vi "THz_TimeDelay.vi"(8 "error in (no error)":errorcluster, 11 "Transport":refnum<class "SMO.Transport.lvclass">) -> (0 "error out":errorcluster, 3 "Transport out":refnum<class "SMO.Transport.lvclass">)   [LabVIEW 2019, in "SMO.Transport.lvclass"]
uses:
  SMO.Transport.lvclass
  <userlib>/LevyLab/Instrument Framework/Instrument Types/Cryostat/Instrument.Cryostat.lvclass
  Control Experiment/Control Experiment.lvclass
  <userlib>/LevyLab/Krohn Hite 7008/Instrument.KH7008.lvclass
  <userlib>/LevyLab/Lockin-Multichannel/Instrument.Lockin/Instrument.Lockin.lvclass
  Control Experiment/Typedefs/Instruments--cluster.ctl
  <userlib>/LevyLab/Instrument Framework/Instrument Types/VSource/Instrument.VSource.lvclass
  <userlib>/LevyLab/Instrument Framework/Instrument Types/VNA/Instrument.VNA.lvclass
  <userlib>/LevyLab/Instrument Framework/Instrument Types/Strain/Instrument.Strain.lvclass
  <userlib>/LevyLab/Instrument Framework/Instrument Types/CBridge/Instrument.CBridge.lvclass
  <vilib>/measure/NI_MAPro.lvlib
  <userlib>/LevyLab/XY Utilities/xy_utilities.lvlib
  <userlib>/LevyLab/XY Utilities/subVIs/Waveform to XY (single).vi
  <userlib>/LevyLab/XY Utilities/subVIs/Get X and Y (single).vi
  <vilib>/measure/maspectr.llb/FFT Power Spectrum and PSD for 1 Chan.vi
  <vilib>/Waveform/WDTOps.llb/WDT Append Waveforms DBL.vi
  <userlib>/_MGI/Timing/MGI Wait/MGI Wait (U32).vi
  <userlib>/LevyLab/Lockin-Multichannel/Instrument.DAQ/Typedefs/Set State-enum.ctl
  <userlib>/LevyLab/Lockin-Multichannel/Instrument.DAQ/Instrument.DAQ.lvclass
  <userlib>/LevyLab/Instrument Framework/Instrument Types/Delay Line/Instrument.DelayLine.lvclass
  SMO.Control Experiment/SMO.Control Experiment.lvclass
  C:/Program Files (x86)/National Instruments/LabVIEW 2019/user.lib/LevyLab/Instrument Framework/SMOs/Instrument/Instrument.lvclass
  C:/Program Files (x86)/National Instruments/LabVIEW 2019/vi.lib/JKI/JKI SMO/SMO/SMO.lvclass
  <vilib>/measure/maresamp.llb/Resample Pair of Arrays (single shot).vi
panel:
  out "Horizontal Progress Bar":dbl(slide)=0.5013000000000001 scale=-0.5..0.5
  out "Signal vs Time":T1(graph)
  out "Delay vs Time":cluster{"Time":dbl[], "Delay":dbl[]}(graph)
  out "Power Spectrum":cluster{"f0":dbl, "df":dbl, "magnitude":dbl[]}[](graph) caption="Power spectrum of time domain signal"
  in  "stop":bool
  in  "Experiment Comments":string="describe only the experiment you're doing right now"
  in  "Experiment Folder":string="05 - folder name"
  out "Delay (ps)":dbl
  out "Elapsed Time (s)":u32
  out "T (mK)":dbl
  out "Refresh Time (ms)":u32
  in  "Sweep Time (s)":dbl=10.0 format="%#_3p"
  in  "Initial Wait (s)":u32=1
  in  "Delay End (ps)":dbl=0.5
  in  "Delay Start (ps)":dbl=-0.5
  in  "Fs (S/s)":dbl=1000.0 min=1000.0 max=204800.0 format="%#_13g"
  in  "Lockin Refresh (s)":dbl=2.0
  in  "Timeout (ms)":i32=1000
  out "Current State":string="Exit"
  # "Start"
  # "End"
  # "*** Folder and comments are only read if this VI is top level. If is is called from Sweep Control then the folder and comments come from Sweep Control.vi ***"
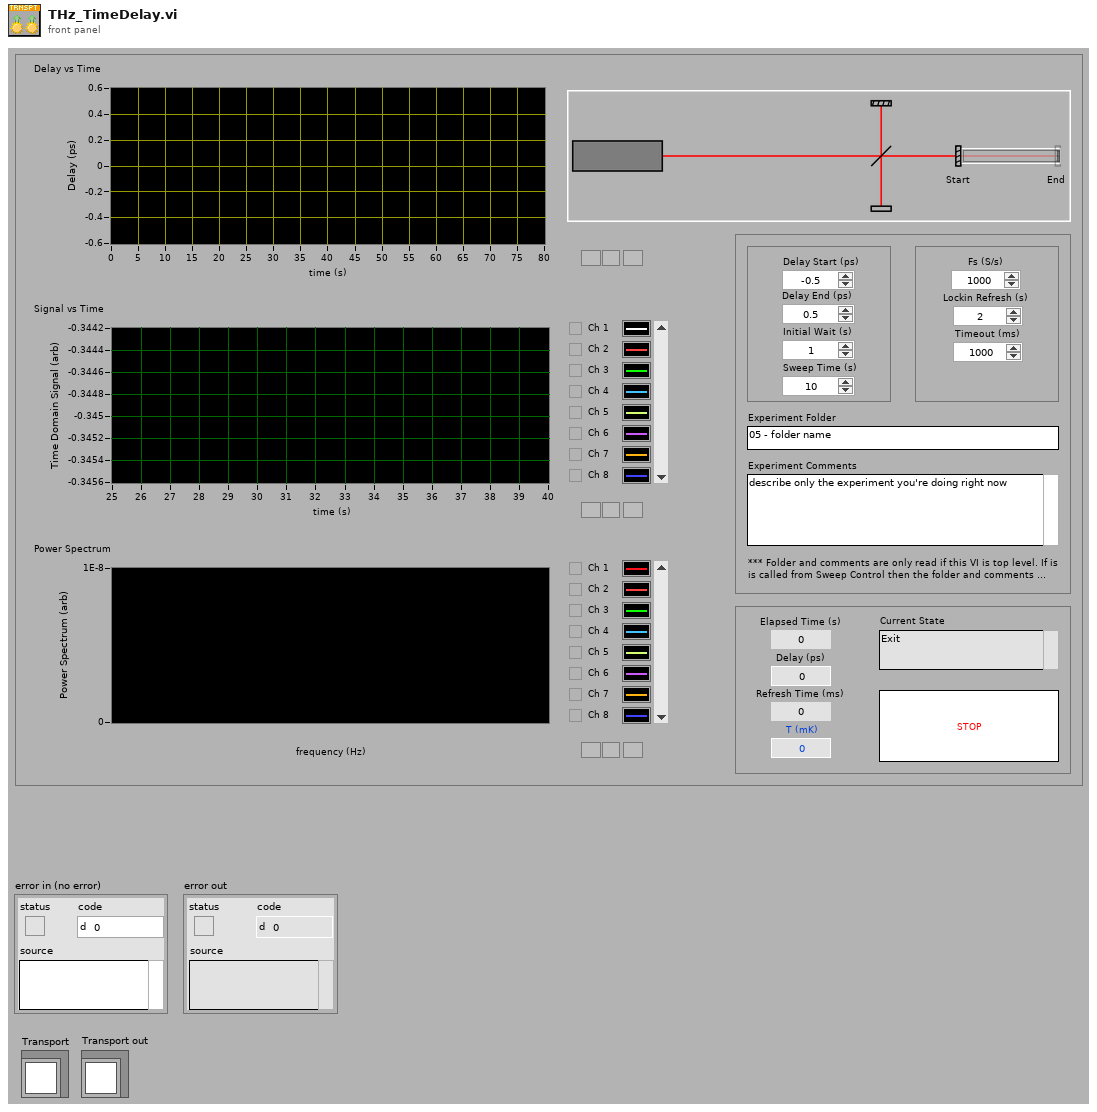
[diagram p1: front panel]
types:
  T1 = cluster{"Delay Start (ps)":dbl, dbl, "Y":dbl[]}[]
  T2 = enum32{"Invalid", "Standard", "Closed", "Hidden", "Minimized", "Maximized"}
  T3 = enum32{"invalid app kind", "Development System", "Run Time System", "Student Edition", "Embedded LabVIEW", "Evaluation", "Custom"}
  T4 = typedef "Lockin.DAQ.lvclass/State-enum.ctl" = enum16{"idle", "created", "started", "stopped", "sweeping"}
  T5 = typedef "Control Experiment.lvclass/Instruments--cluster.ctl" = cluster{"KH7008":refnum<class "Instrument.KH7008.lvclass">[], "Lockin":refnum<class "Instrument.Lockin.lvclass">, "Temperature":refnum<class "Instrument.Cryostat.lvclass">, "Magnet":refnum<class "Instrument.Cryostat.lvclass">, "Rotator":refnum<class "Instrument.Cryostat.lvclass">, "Level":refnum<class "Instrument.Cryostat.lvclass">, "Capacitance Bridge":refnum<class "Instrument.CBridge.lvclass">, "Delay Line":refnum<class "Instrument.DelayLine.lvclass">, "Strain Cell":refnum<class "Instrument.Strain.lvclass">, "VNA":refnum<class "Instrument.VNA.lvclass">, "Voltage Source":refnum<class "Instrument.VSource.lvclass">}
  T6 = cluster{"Core":cluster{"Current VI Reference":refnum<vi>, "Close Panel on Exit?":bool}, "Transport":refnum<class "SMO.Transport.lvclass">, "Control Experiment":refnum<class "SMO.Control Experiment.lvclass">, "Instruments":T5, "Elapsed Time":dbl[], "Absolute Time":dbl[], "Temperature":dbl, "Magnet":dbl, "Delay":dbl[], "AI Waveform (s)":waveform(dbl)[], "AI Waveform (ps)":waveform(dbl)[], "t0":timestamp, "Sweep Value":dbl[], "ms [0]":u32, "ms [i]":u32, "Delay Range (ps)":dbl, "Delay Speed (ps/s)":dbl, "reset":bool, "delay line finish?":bool, "Execution:State":enum32{"Bad", "Idle", "Run top level", "Running"}}
  T7 = enum32{"Bad", "Idle", "Run top level", "Running"}
  T8 = cluster{"Current VI Reference":refnum<vi>, "Close Panel on Exit?":bool}
  T9 = typedef "Instrument.DAQ.lvclass/Get State-enum.ctl" = enum16{"idle", "created", "started", "stopped", "sweeping"}
  T10 = typedef "Instrument.DAQ.lvclass/DAQ.Sampling.Sampling--Cluster.ctl" = cluster{"Fs":dbl, "#s":i32}
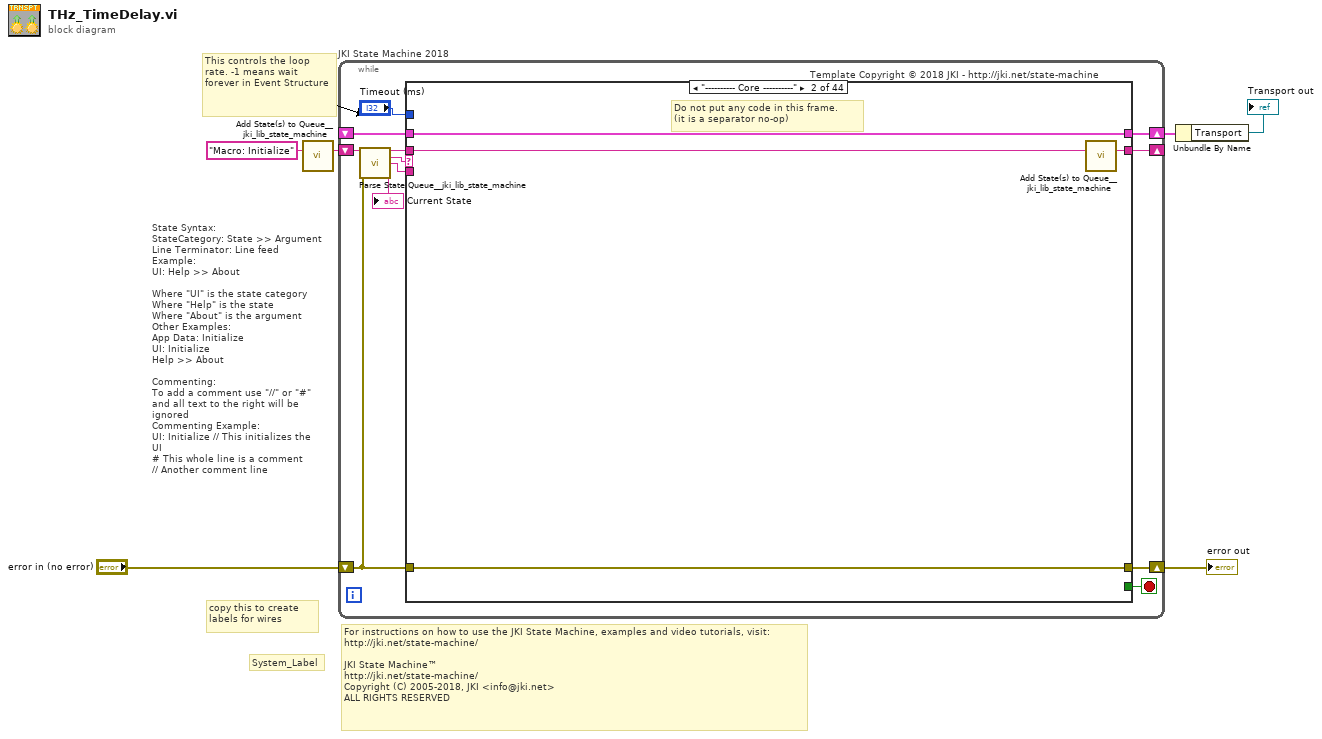
[diagram p0: block diagram]
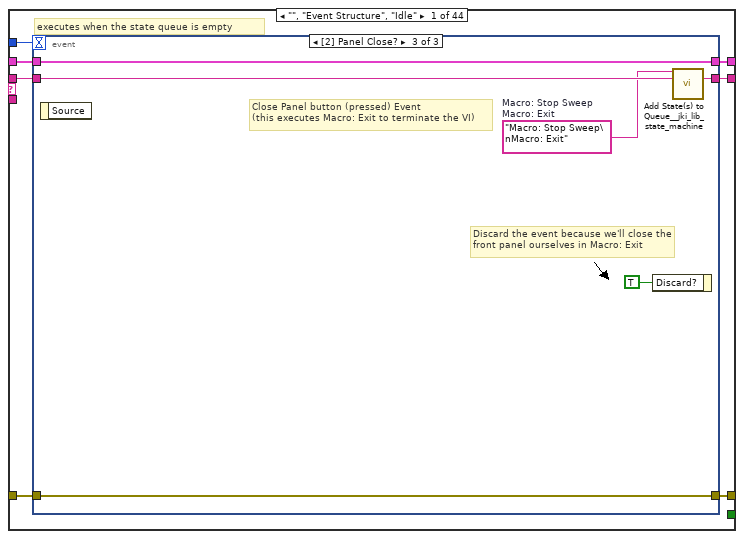
[diagram p2: hidden frame]
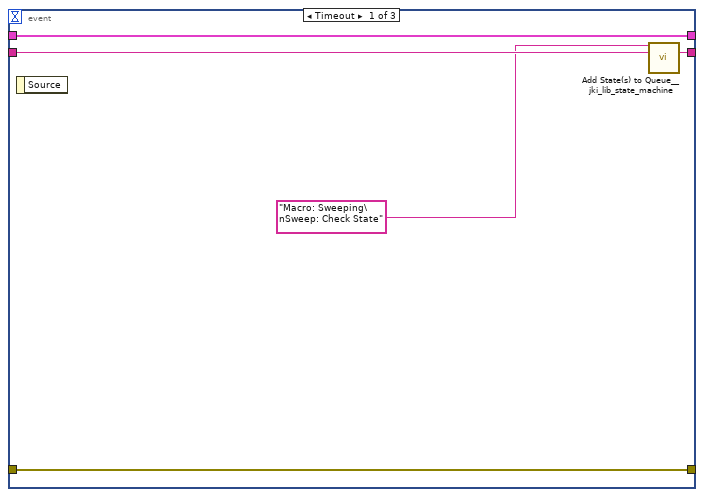
[diagram p3: hidden frame]
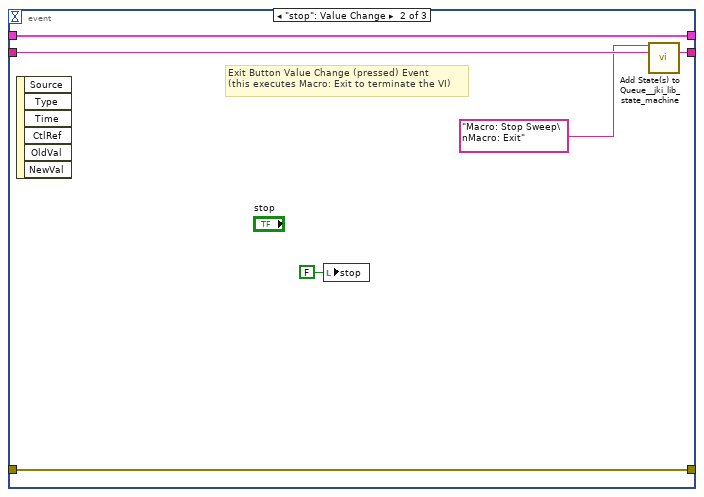
[diagram p4: hidden frame]
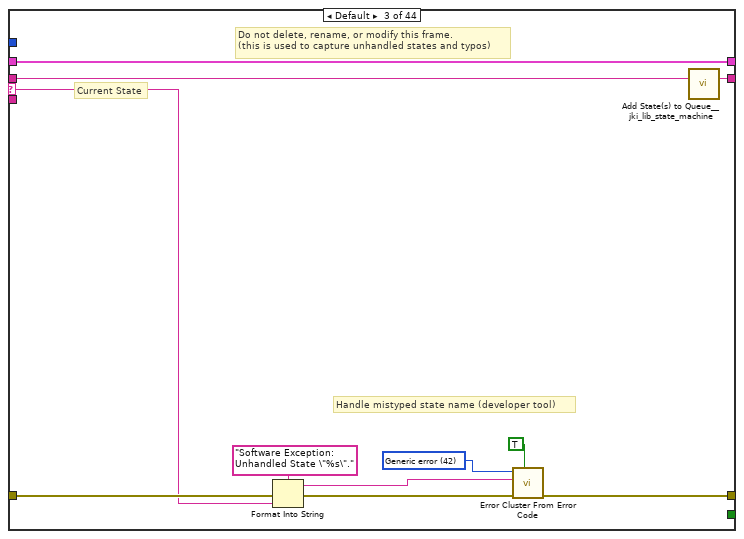
[diagram p5: hidden frame]
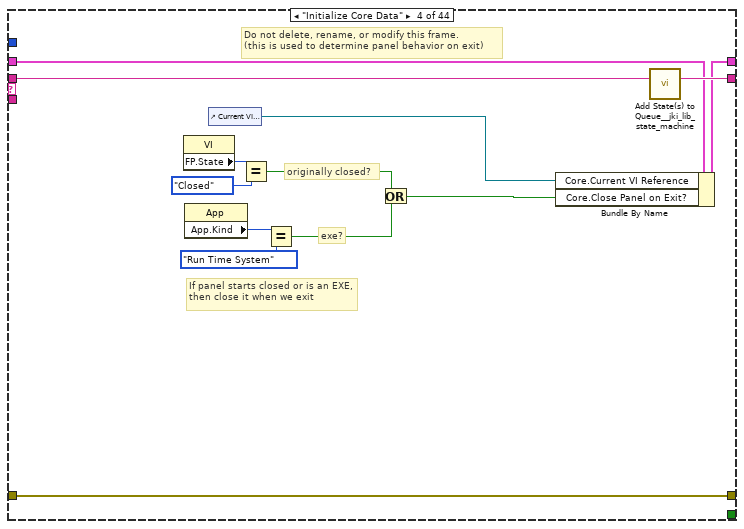
[diagram p6: hidden frame]
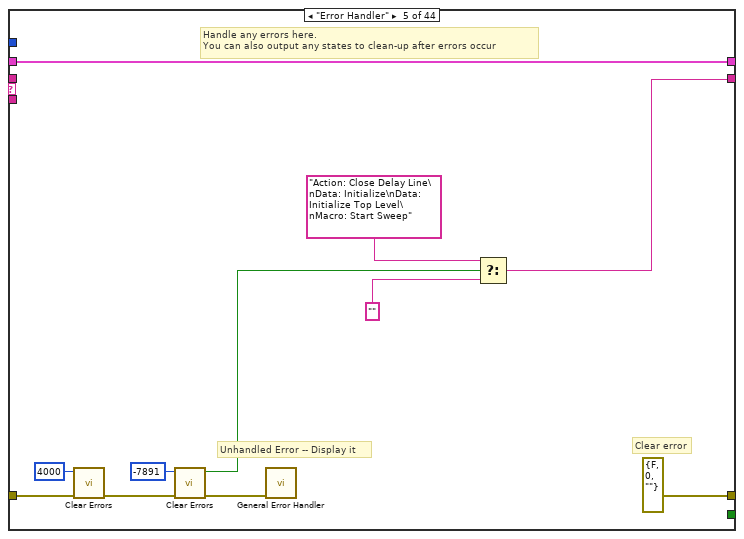
[diagram p7: hidden frame]
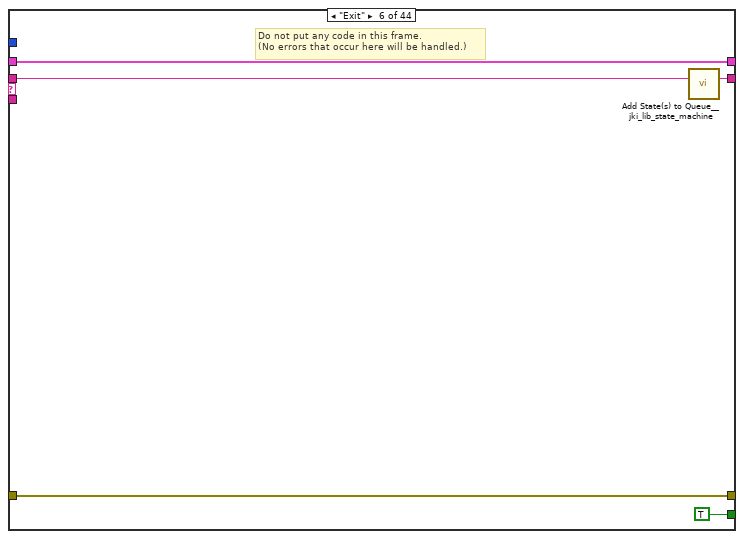
[diagram p8: hidden frame]
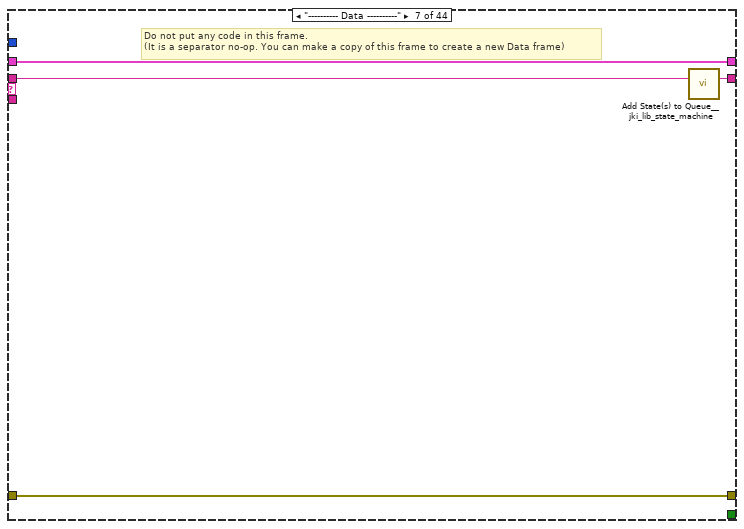
[diagram p9: hidden frame]
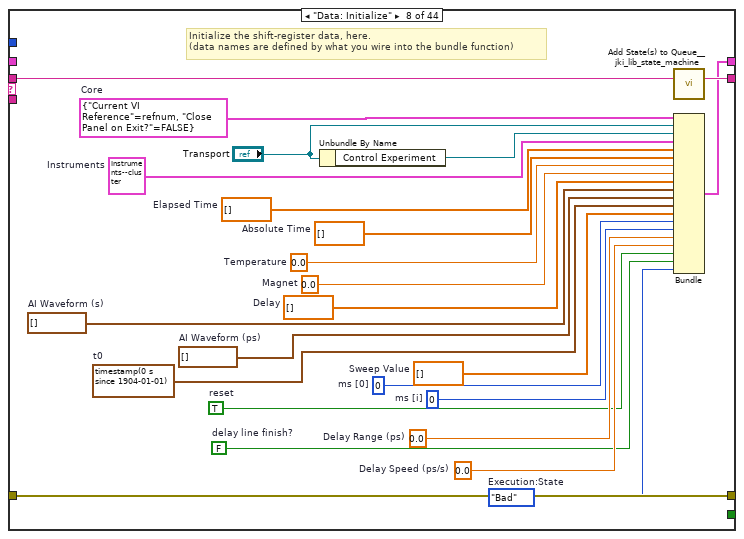
[diagram p10: hidden frame]
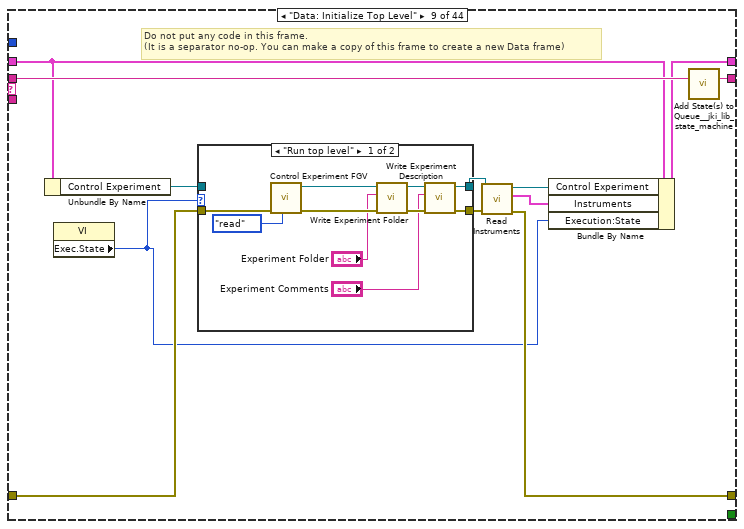
[diagram p11: hidden frame]
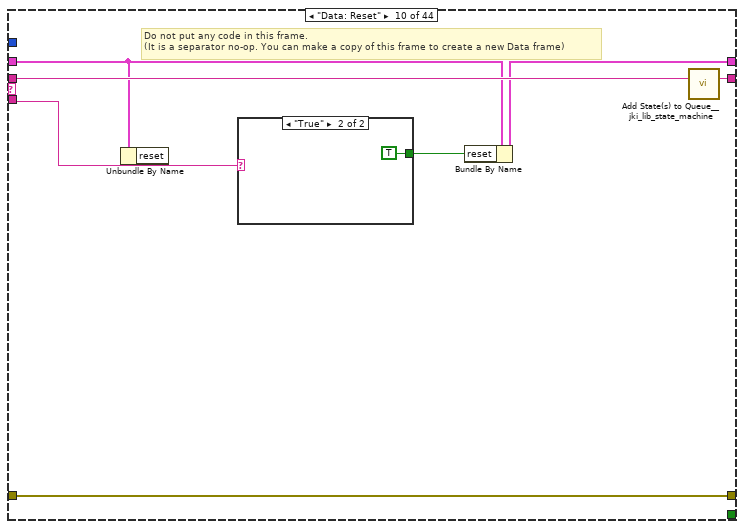
[diagram p13: hidden frame]
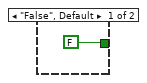
[diagram p14: hidden frame]
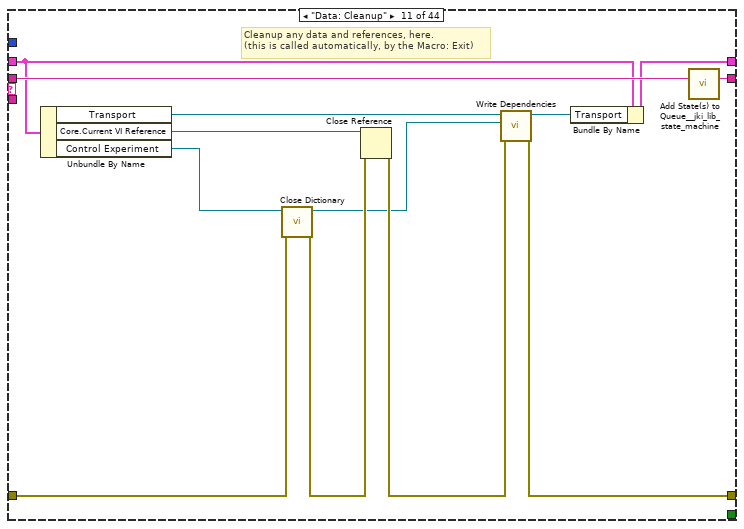
[diagram p15: hidden frame]
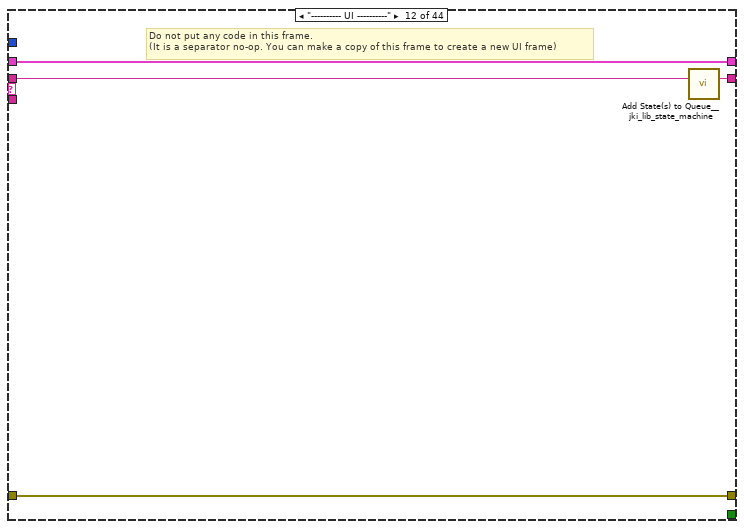
[diagram p16: hidden frame]
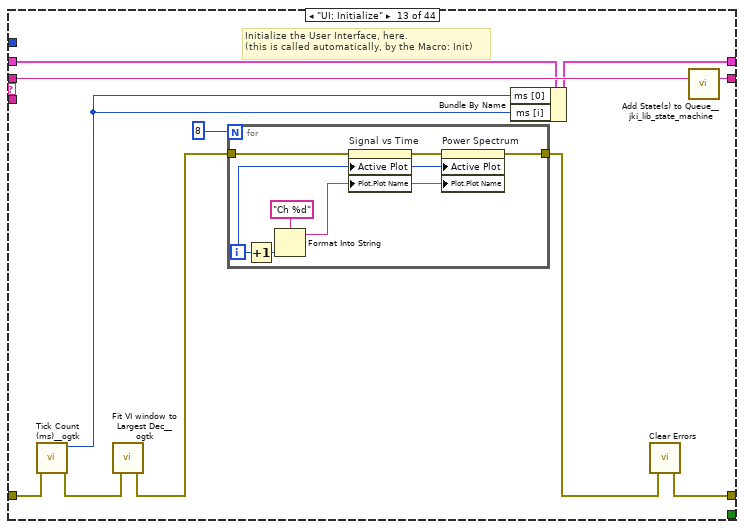
[diagram p17: hidden frame]
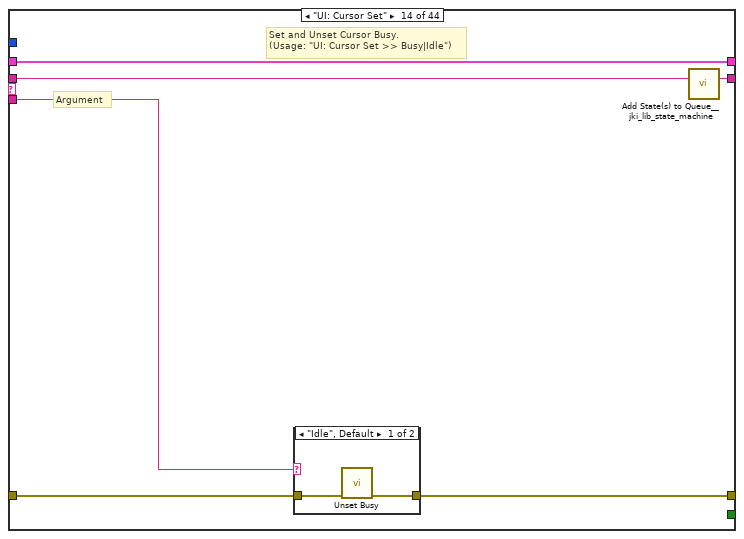
[diagram p18: hidden frame]
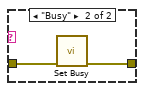
[diagram p19: hidden frame]
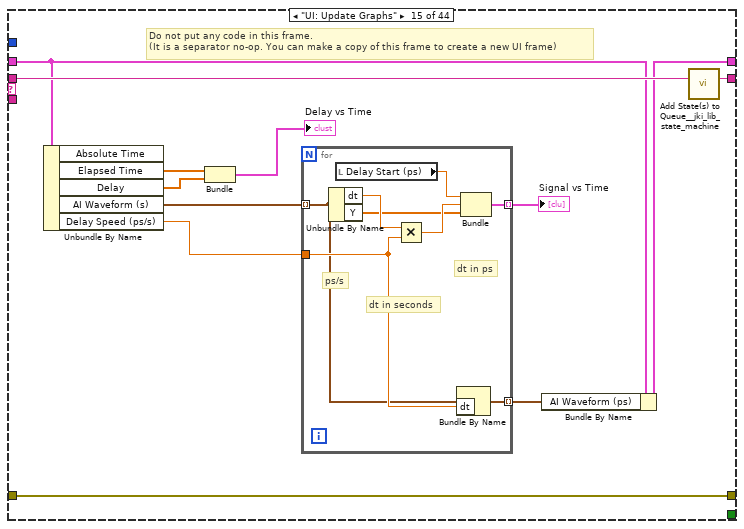
[diagram p20: hidden frame]
diagram:
  # "For instructions on how to use the JKI State Machine, examples and video tutorials, visit:\nhttp://jki.net/state-machine/\n\nJKI State Machine™\nhttp://jki.net/state-machine/\nCopyright (C) 2005-2018, JKI <info@jki.net>\nALL RIGHTS RESERVED"
  # "State Syntax:\nStateCategory: State >> Argument\nLine Terminator: Line feed\nExample:\nUI: Help >> About\n\nWhere \"UI\" is the state category\nWhere \"Help\" is the state\nWhere \"About\" is the argument\nOther Examples:\nApp Data: Initialize\nUI: Initialize\nHelp >> About\n\nCommenting:\nTo add a comment use \"//\" or \"#\" and all text to the right will be ignored\nCommenting Example:\nUI: Initialize // This initializes the UI\n# This whole line is a comment\n// Another comment line"
  # "copy this to create labels for wires"
  # "This controls the loop rate. -1 means wait forever in Event Structure"
  # "System_Label"
  n1 = call <vilib>:"Add State(s) to Queue__jki_lib_state_machine.vi"("State(s) in (\"\")"="Macro: Initialize") -> ("States Out"=w6:string)  [unwired: 14 in]
  n2 = while "JKI State Machine 2018" {
    shift-right: [w11] -> w4
    shift-left: _ -> [w10]
    shift-right: [w14] -> w3
    shift-left: "error in (no error)" -> [w8]
    shift-right: [w13] -> _
    shift-left: w6 -> [w15]
    stop <- w12 stop-if-true
    # "Template Copyright © 2018 JKI - http://jki.net/state-machine"
    n3 = call <vilib>:"Parse State Queue__jki_lib_state_machine.vi"("State Queue"=w15, "Error In (no error)"=w8) -> ("Remaining States"=w17:string, "Current State"=w7:string, "Arguments"=w16:string)  [unwired: 11 in]
    "Current State" <- w7
    n4 = case shown="\"---------- Core ----------\"" w7 {
      selector: w7 -> [_ _ w46 _ _ _ _ _ _ _ _ _ _ _ _ _ _ _ _ _ _ _ _ _ _ _ _ _ _ _ _ _ _ _ _ _ _ _ _ _ _ _ _ _]
      tunnel: w17 -> [w24 w45 w50 w69 _ w85 w89 w113 w125 w144 w159 w163 w174 w187 w203 w226 w244 w251 w320 w328 w333 w338 w343 w353 w357 w371 w379 w383 w391 w396 w415 w422 w467 w482 w492 w496 w508 w563 w585 w602 w606 w610 w624 w669]
      tunnel: w16 -> [_ _ _ _ _ _ _ _ _ w139 _ _ _ w182 _ _ _ w245 _ _ _ _ _ _ _ _ _ _ _ _ _ w420 _ w478 _ _ w497 _ _ _ _ _ _ _]
      tunnel: w10 -> [w22 w42 w48 w62 w79 w83 w86 _ w117 w141 w154 w160 w170 w185 w194 w216 w239 w247 w317 w326 w329 w335 w340 w350 w354 w369 w377 w381 w389 w393 w412 w416 w464 w479 w490 w493 w506 w559 w582 w600 w603 w607 w614 w667]
      tunnel: [w21 w43 w52 w66 errorcluster {"status"=FALSE, "code"=0, "source"=""} ("error out") w82 w87 w110 w118 w142 w148 w161 w164 w183 w200 w218 w234 w248 w318 w325 w331 w336 w341 w351 w355 w362 w375 w380 w384 w394 w413 w417 w465 w473 w487 w494 w502 w553 w577 w591 w604 w608 w620 w666] -> w14
      tunnel: w8 -> [w20 w43 w51 w66 w77 w82 w87 w110 w119 w142 w156 w161 w171 w184 w200 w219 w241 w249 w318 w325 w331 w336 w341 w351 w355 w366 w376 w380 w384 w394 w413 w418 w456 w474 w488 w494 w498 w560 w578 w592 w604 w608 w619 w666]
      tunnel: [w23 w44 w49 w68 w74 w84 w88 w112 w124 w143 w158 w162 w173 w186 w202 w225 w243 w250 w319 w327 w332 w337 w342 w352 w356 w370 w378 w382 w390 w395 w414 w421 w466 w481 w491 w495 w507 w562 w584 w601 w605 w609 w623 w668] -> w13
      tunnel: [_ _ _ _ _ TRUE _ _ _ _ _ _ _ _ _ _ _ _ _ _ _ _ _ _ _ _ _ _ _ _ _ _ _ _ _ _ _ _ _ _ _ _ _ _] -> w12
      tunnel: [w19 w42 w48 w67 w79 w83 w86 w111 w116 w140 w153 w160 w169 w185 w193 w216 w238 w247 w317 w326 w329 w335 w340 w350 w354 w368 w377 w381 w389 w393 w412 w416 w464 w479 w490 w493 w505 w558 w583 w599 w603 w607 w613 w667] -> w11
      tunnel: "Timeout (ms)" -> [w18 _ _ _ _ _ _ _ _ _ _ _ _ _ _ _ _ _ _ _ _ _ _ _ _ _ _ _ _ _ _ _ _ _ _ _ _ _ _ _ _ _ _ _]
      frame "", "Event Structure", "Idle" {
        # "executes when the state queue is empty"
        n5 = event shown="[2] Panel Close?" {
          selector: _ -> [_ _ _]
          dyn-events: _ -> [_ _ _]
          timeout: w18 -> [_ _ _]
          tunnel: w24 -> [w29 w35 w41]
          tunnel: [w28 w34 w40] -> w23
          tunnel: w22 -> [w26 w32 w38]
          tunnel: [w27 w33 w39] -> w21
          tunnel: w20 -> [w27 w33 w39]
          tunnel: [w26 w32 w38] -> w19
          event Timeout {
            n6 = event-data() -> ()  [unwired: 1 in, 1 out]
            n7 = call <vilib>:"Add State(s) to Queue__jki_lib_state_machine.vi"("State(s) in Front (\"\")"="Macro: Sweeping\nSweep: Check State" ("State(s) in Front (\"\")"), "State(s) in (\"\")"=w29) -> ("States Out"=w28:string)  [unwired: 13 in]
          }
          event "stop": Value Change {
            # "Exit Button Value Change (pressed) Event\n(this executes Macro: Exit to terminate the VI)"
            n8 = event-data() -> ()  [unwired: 1 in, 6 out]
            n9 = local write "stop"(FALSE ("stop")) -> ()
            n10 = call <vilib>:"Add State(s) to Queue__jki_lib_state_machine.vi"("State(s) in Front (\"\")"="Macro: Stop Sweep\nMacro: Exit", "State(s) in (\"\")"=w35) -> ("States Out"=w34:string)  [unwired: 13 in]
          }
          event Panel Close? {
            w37 = "Macro: Stop Sweep\nMacro: Exit"  # Macro: Stop Sweep Macro: Exit
            # "Discard the event because we'll close the front panel ourselves in Macro: Exit"
            # "Close Panel button (pressed) Event\n(this executes Macro: Exit to terminate the VI)"
            n11 = event-data() -> ()  [unwired: 1 in, 1 out]
            n12 = event-data("Discard?"=TRUE) -> ()  [unwired: 1 in, 1 out]
            n13 = call <vilib>:"Add State(s) to Queue__jki_lib_state_machine.vi"("State(s) in Front (\"\")"=w37, "State(s) in (\"\")"=w41) -> ("States Out"=w40:string)  [unwired: 13 in]
          }
        }
      }
      frame "---------- Core ----------" {
        # "Do not put any code in this frame.\n(it is a separator no-op)"
        n14 = call <vilib>:"Add State(s) to Queue__jki_lib_state_machine.vi"("State(s) in (\"\")"=w45) -> ("States Out"=w44:string)  [unwired: 14 in]
      }
      frame Default {
        w55 = 42 items=["No error", "Argument error", "Memory is full", "Out of zone", "End of file", "File already open", "Generic file I/O error", "File not found", "File permission error", "Disk is full", "Duplicate path", "Too many files open", "System feature not enabled", "Resource file not found", "Cannot add resource", "Resource not found", "Image not found", "Image memory error", "Pen does not exist", "Config type invalid", "Config token not found", "Config parse error", "Config memory error", "Bad external code format", "Bad external code offset", "External code not present", "Null window", "Destroy window error", "Null menu", "Print aborted", "Bad print record", "Print driver error", "Windows error during printing", "Memory error during printing", "Print dialog error", "Generic print error", "Invalid device refnum", "Device not found", "Device parameter error", "Device unit error", "Cannot open device", "Device call aborted", "Generic error", "Cancelled by user", "Object ID too low", "Object ID too high", "Object not in heap", "Unknown heap", "Unknown object (invalid DefProc)", "Unknown object (DefProc not in table)", "Message out of range", "Invalid (null) method", "Unknown message", "Manager call not supported", "Bad address", "Network operation in progress", "Network operation timed out", "Connection is busy", "Network attribute not supported", "Network error", "Address in use", "System out of memory", "Connection aborted", "Connection refused", "Not connected", "Already connected", "Connection closed", "Initialization error (interapplication manager)", "Bad occurrence", "Wait on unbound occurrence handler", "Occurrence queue overflow", "Datalog type conflict", "Unused", "Unrecognized type (interapplication manager)", "Memory corrupt", "Failed to make temporary DLL", "Old CIN version", "Drag socket not found", "Failed to load drop-object", "Failed to register OLE object", "Failed to release OLE object", "Format specifier type mismatch", "Unknown format specifier", "Too few format specifiers", "Too many format specifiers", "Scan failed", "Newer CIN version", "Error converting to variant", "Runtime menu error", "Password tampered", "Variant attribute not found", "Incompatible variant data type", "Event data is not available", "Event Store is not present", "Occurrence is not found", "Event Queue is not created", "Event info is not available", "Refnum passed is NULL", "Error retrieving Class GUID", "Error retrieving CoClass GUID", "Error retrieving TypeLib GUID.", "Bad built application magic bytes.", "Specific driver is different from the specific driver associated with the Logical Name.", "There is no session opened to the class driver.", "Max Error", "MAX - Error with config objects", "MAX - Error loading configuration", "MAX - Group not supported"]
        # "Current State"
        # "Do not delete, rename, or modify this frame.\n(this is used to capture unhandled states and typos)"
        # "Handle mistyped state name (developer tool)"
        n15 = Format Into String(format string="Software Exception: Unhandled State \"%s\"." ("message"), error in=w51, w46) -> (resulting string=w54:string, error out=w53:errorcluster)  [unwired: 1 in]
        n16 = call <vilib>:"Error Cluster From Error Code.vi"("show call chain? (False)"=TRUE, "error in (no error)"=w53, "error message (\"\")"=w54, "error code (0)"=w55) -> ("error out"=w52:errorcluster)  [unwired: 5 in]
        n17 = call <vilib>:"Add State(s) to Queue__jki_lib_state_machine.vi"("State(s) in (\"\")"=w50) -> ("States Out"=w49:string)  [unwired: 14 in]
      }
      frame "Initialize Core Data" {
        # "Do not delete, rename, or modify this frame.\n(this is used to determine panel behavior on exit)"
        # "originally closed?"
        # "exe?"
        # "If panel starts closed or is an EXE, then close it when we exit"
        n18 = property class="VI"() -> ("FP.State"=w59:T2)  [unwired: 2 in, 2 out]
        n19 = property class="App"() -> ("App.Kind"=w65:T3)  [unwired: 2 in, 2 out]
        n20 = control-ref of="Current VI Reference"() -> (w60:refnum<vi>)
        n21 = Equal?(x=w59, y=T2."Closed" ("Front Panel Window:State")) -> (x = y?=w57:bool)
        n22 = Equal?(x=w65, y=T3."Run Time System" ("Application:Kind")) -> (x = y?=w63:bool)
        n23 = Or(x=w57, y=w63) -> (x .or. y?=w61:bool)
        n24 = Bundle By Name(cluster=w62, "Core.Current VI Reference"=w60, "Core.Close Panel on Exit?"=w61) -> (w67:T6)
        n25 = call <vilib>:"Add State(s) to Queue__jki_lib_state_machine.vi"("State(s) in (\"\")"=w69) -> ("States Out"=w68:string)  [unwired: 14 in]
      }
      frame "Error Handler" {
        # "Unhandled Error -- Display it"
        # "Handle any errors here.\nYou can also output any states to clean-up after errors occur"
        # "Clear error"
        n26 = call <vilib>:"Clear Errors.vi"("error in (no error)"=w77, "specific error code to clear (0: all)"=4000) -> ("error out"=w72:errorcluster)  [unwired: 4 in, 1 out]
        n27 = call <vilib>:"Clear Errors.vi"("error in (no error)"=w72, "specific error code to clear (0: all)"=-7891) -> ("error out"=w71:errorcluster, "specific error cleared?"=w70:bool)  [unwired: 4 in]
        n28 = call <vilib>:"General Error Handler.vi"("error in (no error)"=w71) -> ()  [unwired: 10 in, 5 out]
        n29 = Select(t="Action: Close Delay Line\nData: Initialize\nData: Initialize Top Level\nMacro: Start Sweep", s=w70, f="") -> (s? t:f=w74:string)
      }
      frame "Exit" {
        # "Do not put any code in this frame.\n(No errors that occur here will be handled.)"
        n30 = call <vilib>:"Add State(s) to Queue__jki_lib_state_machine.vi"("State(s) in (\"\")"=w85) -> ("States Out"=w84:string)  [unwired: 14 in]
      }
      frame "---------- Data ----------" {
        # "Do not put any code in this frame.\n(It is a separator no-op. You can make a copy of this frame to create a new Data frame)"
        n31 = call <vilib>:"Add State(s) to Queue__jki_lib_state_machine.vi"("State(s) in (\"\")"=w89) -> ("States Out"=w88:string)  [unwired: 14 in]
      }
      frame "Data: Initialize" {
        w90 = T7."Bad"  # Execution:State
        w91 = waveform(dbl)[] []  # AI Waveform (ps)
        w92 = FALSE  # delay line finish?
        w93 = TRUE  # reset
        w98 = dbl[] []  # Absolute Time
        w94 = waveform(dbl)[] []  # AI Waveform (s)
        w100 = timestamp(0 s since 1904-01-01)  # t0
        w101 = 0.0  # Delay Speed (ps/s)
        w95 = dbl[] []  # Delay
        w102 = 0.0  # Delay Range (ps)
        w103 = dbl[] []  # Sweep Value
        w105 = u32 0  # ms [i]
        w106 = u32 0  # ms [0]
        w99 = dbl[] []  # Elapsed Time
        w96 = 0.0  # Magnet
        w97 = 0.0  # Temperature
        w107 = T5 {"KH7008"=[], "Lockin"=refnum, "Temperature"=refnum, "Magnet"=refnum, "Rotator"=refnum, "Level"=refnum, "Capacitance Bridge"=refnum, "Delay Line"=refnum, "Strain Cell"=refnum, "VNA"=refnum, "Voltage Source"=refnum}  # Instruments
        w109 = T8 {"Current VI Reference"=refnum, "Close Panel on Exit?"=FALSE}  # Core
        # "Initialize the shift-register data, here.\n(data names are defined by what you wire into the bundle function)"
        n32 = Unbundle By Name("Transport") -> ("Control Experiment"=w104:refnum<class "SMO.Control Experiment.lvclass">)
        n33 = call <vilib>:"Add State(s) to Queue__jki_lib_state_machine.vi"("State(s) in (\"\")"=w113) -> ("States Out"=w112:string)  [unwired: 14 in]
        n34 = Bundle("Core"=w109, "Transport"="Transport", "Control Experiment"=w104, "Instruments"=w107, "Elapsed Time"=w99, "Absolute Time"=w98, "Temperature"=w97, "Magnet"=w96, "Delay"=w95, "AI Waveform (s)"=w94, "AI Waveform (ps)"=w91, "t0"=w100, "Sweep Value"=w103, "ms [0]"=w106, "ms [i]"=w105, "Delay Range (ps)"=w102, "Delay Speed (ps/s)"=w101, "reset"=w93, "delay line finish?"=w92, "Execution:State"=w90) -> (w111:T6)  [unwired: 1 in]
      }
      frame "Data: Initialize Top Level" {
        # "Do not put any code in this frame.\n(It is a separator no-op. You can make a copy of this frame to create a new Data frame)"
        n35 = Unbundle By Name(w117) -> ("Control Experiment"=w120:refnum<class "SMO.Control Experiment.lvclass">)
        n36 = property class="VI"() -> ("Exec.State"=w114:T7)  [unwired: 2 in, 2 out]
        n37 = case shown="\"Run top level\"" w114 {
          tunnel: w119 -> [w135 w136]
          tunnel: [w130 w136] -> w121
          tunnel: [w129 w137] -> w122
          tunnel: w120 -> [_ w137]
          frame "Run top level" {
            n38 = call "Control Experiment FGV.vi"("Function"=enum16{"read", "write"}."read", "error in (no error)"=w135) -> ("error out"=w133:errorcluster, "Control Experiment.lvclass out"=w134:refnum<class "Control Experiment.lvclass">)  [unwired: 8 in]
            n39 = call "Write Experiment Folder.vi"("error in (no error)"=w133, "Experiment Folder"="Experiment Folder", "Control Experiment in"=w134) -> ("error out"=w131:errorcluster, "Control Experiment out"=w132:refnum<class "Control Experiment.lvclass">)  [unwired: 7 in]
            n40 = call "Write Experiment Description.vi"("error in (no error)"=w131, "Experiment Description"="Experiment Comments", "Control Experiment in"=w132) -> ("error out"=w130:errorcluster, "Control Experiment out"=w129:refnum<class "Control Experiment.lvclass">)  [unwired: 7 in]
          }
          frame "Running", Default {
          }
        }
        n41 = call "Read Instruments.vi"("error in (no error)"=w121, "Control Experiment in"=w122) -> ("error out"=w118:errorcluster, "Instruments"=w123:T5, "Control Experiment out"=w115:refnum<class "Control Experiment.lvclass">)  [unwired: 7 in]
        n42 = Bundle By Name(cluster=w117, "Control Experiment"=w115, "Instruments"=w123, "Execution:State"=w114) -> (w116:T6)
        n43 = call <vilib>:"Add State(s) to Queue__jki_lib_state_machine.vi"("State(s) in (\"\")"=w125) -> ("States Out"=w124:string)  [unwired: 14 in]
      }
      frame "Data: Reset" {
        # "Do not put any code in this frame.\n(It is a separator no-op. You can make a copy of this frame to create a new Data frame)"
        n44 = Unbundle By Name(w141) -> ()  [unwired: 1 out]
        n45 = case shown="\"True\"" w139 {
          tunnel: [FALSE ("reset") TRUE ("reset")] -> w138
          frame "False", Default {
          }
          frame "True" {
          }
        }
        n46 = Bundle By Name(cluster=w141, "reset"=w138) -> (w140:T6)
        n47 = call <vilib>:"Add State(s) to Queue__jki_lib_state_machine.vi"("State(s) in (\"\")"=w144) -> ("States Out"=w143:string)  [unwired: 14 in]
      }
      frame "Data: Cleanup" {
        # "Cleanup any data and references, here.\n(this is called automatically, by the Macro: Exit)"
        n48 = Unbundle By Name(w154) -> ("Transport"=w151:refnum<class "SMO.Transport.lvclass">, "Core.Current VI Reference"=w157:refnum<vi>, "Control Experiment"=w150:refnum<class "SMO.Control Experiment.lvclass">)
        n49 = call "Close Dictionary.vi"("error in (no error)"=w156, "Control Experiment in"=w150) -> ("error out"=w155:errorcluster, "Control Experiment out"=w147:refnum<class "Control Experiment.lvclass">)  [unwired: 8 in]
        n50 = Close Reference(reference=w157, error in (no error)=w155) -> (error out=w149:errorcluster)
        n51 = call "Write Dependencies.vi"("error in (no error)"=w149, "Control Experiment"=w147, "Transport in"=w151) -> ("error out"=w148:errorcluster, "Transport out"=w152:refnum<class "SMO.Transport.lvclass">)  [unwired: 7 in]
        n52 = Bundle By Name(cluster=w154, "Transport"=w152) -> (w153:T6)
        n53 = call <vilib>:"Add State(s) to Queue__jki_lib_state_machine.vi"("State(s) in (\"\")"=w159) -> ("States Out"=w158:string)  [unwired: 14 in]
      }
      frame "---------- UI ----------" {
        # "Do not put any code in this frame.\n(It is a separator no-op. You can make a copy of this frame to create a new UI frame)"
        n54 = call <vilib>:"Add State(s) to Queue__jki_lib_state_machine.vi"("State(s) in (\"\")"=w163) -> ("States Out"=w162:string)  [unwired: 14 in]
      }
      frame "UI: Initialize" {
        # "Initialize the User Interface, here.\n(this is called automatically, by the Macro: Init)"
        n55 = call <userlib>:"Tick Count (ms)__ogtk.vi"("error in (no error)"=w171) -> ("error out"=w167:errorcluster, "millisecond timer value"=w168:u32)  [unwired: 9 in]
        n56 = call <userlib>:"Fit VI window to Largest Dec__ogtk.vi"("error in (no error)"=w167) -> ("error out"=w166:errorcluster)  [unwired: 5 in, 1 out]
        n57 = for {
          N: 8 -> [_]
          tunnel: w166 -> [w180]
          tunnel: [w176] -> w165
          i -> [w177]
          n58 = Increment(x=w177) -> (x+1=w179:i32)
          n59 = Format Into String(format string="Ch %d", w179) -> (resulting string=w175:string)  [unwired: 2 in, 1 out]
          n60 = property on="Signal vs Time" class="WFGraph (strict)"(error in=w180, "Active Plot"=w177, "Plot.Plot Name"=w175) -> (error out=w178:errorcluster)  [unwired: 1 in, 1 out]
          n61 = property on="Power Spectrum" class="WFGraph (strict)"(error in=w178, "Active Plot"=w177, "Plot.Plot Name"=w175) -> (error out=w176:errorcluster)  [unwired: 1 in, 1 out]
        }
        n62 = Bundle By Name(cluster=w170, "ms [0]"=w168, "ms [i]"=w168) -> (w169:T6)
        n63 = call <vilib>:"Clear Errors.vi"("error in (no error)"=w165) -> ("error out"=w164:errorcluster)  [unwired: 5 in, 1 out]
        n64 = call <vilib>:"Add State(s) to Queue__jki_lib_state_machine.vi"("State(s) in (\"\")"=w174) -> ("States Out"=w173:string)  [unwired: 14 in]
      }
      frame "UI: Cursor Set" {
        # "Argument"
        # "Set and Unset Cursor Busy.\n(Usage: \"UI: Cursor Set >> Busy|Idle\")"
        n65 = case shown="\"Idle\", Default" w182 {
          tunnel: w184 -> [w189 w191]
          tunnel: [w188 w190] -> w183
          frame "Idle", Default {
            n66 = call <vilib>:"Unset Busy.vi"("error in (no error)"=w189) -> ("error out"=w188:errorcluster)  [unwired: 10 in]
          }
          frame "Busy" {
            n67 = call <vilib>:"Set Busy.vi"("error in (no error)"=w191) -> ("error out"=w190:errorcluster)  [unwired: 9 in, 1 out]
          }
        }
        n68 = call <vilib>:"Add State(s) to Queue__jki_lib_state_machine.vi"("State(s) in (\"\")"=w187) -> ("States Out"=w186:string)  [unwired: 14 in]
      }
      frame "UI: Update Graphs" {
        # "Do not put any code in this frame.\n(It is a separator no-op. You can make a copy of this frame to create a new UI frame)"
        n69 = Unbundle By Name(w194) -> ("Elapsed Time"=w201:dbl[], "Delay"=w199:dbl[], "AI Waveform (s)"=w197:waveform(dbl)[], "Delay Speed (ps/s)"=w195:dbl)  [unwired: 1 out]
        n70 = Bundle("Elapsed Time"=w201, "Delay"=w199) -> (→"Delay vs Time":cluster{"Elapsed Time":dbl[], "Delay":dbl[]})  [unwired: 1 in]
        n71 = for {
          tunnel: w197 -> [w205] mode=indexing
          tunnel: [w207] -> w196 mode=indexing
          tunnel: w195 -> [w206]
          tunnel: [w204] -> w192 mode=indexing
          # "dt in ps"
          # "ps/s"
          # "dt in seconds"
          n72 = Unbundle By Name(w205) -> ("dt"=w211:dbl, "Y"=w209:dbl[])
          n73 = local read "Delay Start (ps)"() -> (w208:dbl)
          n74 = Multiply(x=w211, y=w206) -> (x*y=w210:dbl)
          n75 = Bundle By Name(cluster=w205, "dt"=w206) -> (w204:waveform(dbl))
          n76 = Bundle("Delay Start (ps)"=w208, w210, "Y"=w209) -> (w207:cluster{"Delay Start (ps)":dbl, dbl, "Y":dbl[]})  [unwired: 1 in]
        }
        "Signal vs Time" <- w196
        n77 = Bundle By Name(cluster=w194, "AI Waveform (ps)"=w192) -> (w193:T6)
        n78 = call <vilib>:"Add State(s) to Queue__jki_lib_state_machine.vi"("State(s) in (\"\")"=w203) -> ("States Out"=w202:string)  [unwired: 14 in]
      }
      frame "UI: Update Graphs Final" {
        # "Do not put any code in this frame.\n(It is a separator no-op. You can make a copy of this frame to create a new UI frame)"
        n79 = Unbundle By Name(w216) -> ("Absolute Time"=w214:dbl[], "Elapsed Time"=w221:dbl[], "Delay"=w215:dbl[], "AI Waveform (s)"=w212:waveform(dbl)[])
        n80 = Index Array(array=w212) -> (element=w224:waveform(dbl))  [unwired: 1 in]
        n81 = Bundle("Elapsed Time"=w221, "Delay"=w215) -> ()  [unwired: 1 in, 1 out]
        n82 = Unbundle By Name(w224) -> ("dt"=w223:dbl, "t0"=w222:timestamp)
        n83 = Bundle("Absolute Time"=w214, "Delay"=w215) -> (w213:cluster{"Absolute Time":dbl[], "Delay":dbl[]})  [unwired: 1 in]
        n84 = To Double Precision Float(number=w222) -> (double precision float=w220:dbl)
        n85 = call-poly <vilib>:"Resample Waveforms (single shot).vi"("XY-data in"=w213, "dt"=w223, "t0"=w220, "error in (no error)"=w219) -> ("resampled waveform out"=w217:waveform(dbl), "error out"=w218:errorcluster)  [unwired: 7 in, 3 out]
        n86 = for {
          tunnel: w217 -> [w231]
          tunnel: w212 -> [w230] mode=indexing
          tunnel: [w227] -> _ mode=indexing
          n87 = Unbundle By Name(w231) -> ("Y"=w229:dbl[])
          n88 = Unbundle By Name(w230) -> ("Y"=w228:dbl[])
          n89 = Bundle("Y"=w229, "Y"=w228) -> (w227:cluster{"Y":dbl[], "Y":dbl[]})  [unwired: 1 in]
        }
        n90 = call <vilib>:"Add State(s) to Queue__jki_lib_state_machine.vi"("State(s) in (\"\")"=w226) -> ("States Out"=w225:string)  [unwired: 14 in]
      }
      frame "UI: Update Timer" {
        n91 = Unbundle By Name(w239) -> ("ms [0]"=w240:u32)
        n92 = call <userlib>:"Tick Count (ms)__ogtk.vi"("error in (no error)"=w241) -> ("error out"=w235:errorcluster, "millisecond timer value"=w233:u32)  [unwired: 9 in]
        n93 = Subtract(x=w233, y=w240) -> (x-y=w237:u32)
        n94 = call <userlib>:"MGI Milliseconds Since Last Call.vi"("Error In"=w235) -> ("ms"=→"Refresh Time (ms)":u32, "Error Out"=w234:errorcluster)  [unwired: 5 in]
        n95 = Divide(x=w237, y=u32 1000 ("x")) -> (x/y=→"Elapsed Time (s)":dbl)
        n96 = Bundle By Name(cluster=w239, "ms [i]"=w233) -> (w238:T6)
        n97 = call <vilib>:"Add State(s) to Queue__jki_lib_state_machine.vi"("State(s) in (\"\")"=w244) -> ("States Out"=w243:string)  [unwired: 14 in]
      }
      frame "UI: Front Panel State" {
        # "Argument"
        # "Set Front Panel Open or Closed\n(Usage: \"UI: Front Panel State >> Open|Close\")"
        n98 = Unbundle By Name(w247) -> ("Core.Current VI Reference"=w246:refnum<vi>)
        n99 = case shown="\"Open\", \"Standard\", Default" w245 {
          tunnel: w249 -> [w257 w272 w283 w296 w309]
          tunnel: [w259 w273 w285 w298 w311] -> w248
          tunnel: w246 -> [w258 w270 w284 w297 w310]
          frame "Open", "Standard", Default {
            w252 = T2."Standard" ("State")
            n100 = property class="VI"(reference=w258, error in=w257) -> (reference out=w255:refnum<vi>, error out=w256:errorcluster, "FP.State"=w254:T2)
            n101 = Not Equal?(x=w254, y=w252) -> (x != y?=w253:bool)
            n102 = case shown="False" w253 {
              tunnel: [w263 w265] -> w259
              tunnel: w256 -> [w262 w265]
              tunnel: w255 -> [w261 _]
              tunnel: w252 -> [w260 _]
              frame True {
                n103 = invoke class="VI" method="FP.Open"(reference=w261, error in=w262, "Activate"=TRUE, "State"=w260) -> (error out=w263:errorcluster)  [unwired: 1 in, 4 out]
              }
              frame False {
              }
            }
          }
          frame "Close", "Closed" {
            n104 = property class="VI"(reference=w270, error in=w272) -> (reference out=w269:refnum<vi>, error out=w271:errorcluster, "FP.State"=w267:T2)
            n105 = Not Equal?(x=w267, y=T2."Closed" ("Front Panel Window:State")) -> (x != y?=w266:bool)
            n106 = case shown="True" w266 {
              tunnel: [w274 w277] -> w273
              tunnel: w271 -> [w274 w276]
              tunnel: w269 -> [_ w275]
              frame False {
              }
              frame True {
                n107 = invoke class="VI" method="FP.Close"(reference=w275, error in=w276) -> (error out=w277:errorcluster)  [unwired: 1 in, 2 out]
              }
            }
          }
          frame "Hidden", "Hide" {
            w278 = T2."Hidden" ("State")
            n108 = property class="VI"(reference=w284, error in=w283) -> (reference out=w281:refnum<vi>, error out=w282:errorcluster, "FP.State"=w280:T2)
            n109 = Not Equal?(x=w280, y=w278) -> (x != y?=w279:bool)
            n110 = case shown="True" w279 {
              tunnel: [w289 w290] -> w285
              tunnel: w282 -> [w288 w290]
              tunnel: w281 -> [w287 _]
              tunnel: w278 -> [w286 _]
              frame True {
                n111 = invoke class="VI" method="FP.Open"(reference=w287, error in=w288, "State"=w286) -> (error out=w289:errorcluster)  [unwired: 2 in, 4 out]
              }
              frame False {
              }
            }
          }
          frame "Minimize", "Minimized" {
            w291 = T2."Minimized" ("State")
            n112 = property class="VI"(reference=w297, error in=w296) -> (reference out=w294:refnum<vi>, error out=w295:errorcluster, "FP.State"=w293:T2)
            n113 = Not Equal?(x=w293, y=w291) -> (x != y?=w292:bool)
            n114 = case shown="True" w292 {
              tunnel: [w302 w303] -> w298
              tunnel: w295 -> [w301 w303]
              tunnel: w294 -> [w300 _]
              tunnel: w291 -> [w299 _]
              frame True {
                n115 = invoke class="VI" method="FP.Open"(reference=w300, error in=w301, "State"=w299) -> (error out=w302:errorcluster)  [unwired: 2 in, 4 out]
              }
              frame False {
              }
            }
          }
          frame "Maximize", "Maximized" {
            w304 = T2."Maximized" ("State")
            n116 = property class="VI"(reference=w310, error in=w309) -> (reference out=w307:refnum<vi>, error out=w308:errorcluster, "FP.State"=w306:T2)
            n117 = Not Equal?(x=w306, y=w304) -> (x != y?=w305:bool)
            n118 = case shown="True" w305 {
              tunnel: [w315 w316] -> w311
              tunnel: w308 -> [w314 w316]
              tunnel: w307 -> [w313 _]
              tunnel: w304 -> [w312 _]
              frame True {
                n119 = invoke class="VI" method="FP.Open"(reference=w313, error in=w314, "State"=w312) -> (error out=w315:errorcluster)  [unwired: 2 in, 4 out]
              }
              frame False {
              }
            }
          }
        }
        n120 = call <vilib>:"Add State(s) to Queue__jki_lib_state_machine.vi"("State(s) in (\"\")"=w251) -> ("States Out"=w250:string)  [unwired: 14 in]
      }
      frame "---------- Macro ----------" {
        # "Do not put any code in this frame.\n(It is a separator no-op. You can make a copy of this frame to create a new Macro frame)"
        n121 = call <vilib>:"Add State(s) to Queue__jki_lib_state_machine.vi"("State(s) in (\"\")"=w320) -> ("States Out"=w319:string)  [unwired: 14 in]
      }
      frame "Macro: Initialize" {
        w323 = FALSE  # debug mode
        w322 = "Data: Initialize\nInitialize Core Data\nUI: Initialize\nUI: Front Panel State >> Open\nUI: Front Panel State >> Open\nData: Initialize Top Level\nData: Reset >> True\nSweep: Initialize\nSweep: Simulate\nMacro: Exit"  # debug mode
        # "Initialization Macro\n(This is called once, when the VI starts)"
        n122 = Select(t=w322, s=w323, f="Data: Initialize\nInitialize Core Data\nUI: Initialize\nUI: Front Panel State >> Open\nData: Initialize Top Level\nData: Reset >> True\nMacro: Start Sweep\n") -> (s? t:f=w324:string)
        n123 = call <vilib>:"Add State(s) to Queue__jki_lib_state_machine.vi"("State(s) in Front (\"\")"=w324, "State(s) in (\"\")"=w328) -> ("States Out"=w327:string)  [unwired: 13 in]
      }
      frame "Macro: Start Sweep" {
        # "Do not put any code in this frame.\n(It is a separator no-op. You can make a copy of this frame to create a new Macro frame)"
        n124 = call <vilib>:"Add State(s) to Queue__jki_lib_state_machine.vi"("State(s) in Front (\"\")"="Sweep: Initialize\nAction: Move Delay Line >> Start\n//Action: Lockin >> Stop\nAction: Lockin Sampling\nSweep: Wait\nMeasure: Lockin >> Start\n//Action: Lockin >> Start\nMeasure: Delay Line\nAction: Move Delay Line >> End" ("State(s) in Front (\"\")"), "State(s) in (\"\")"=w333) -> ("States Out"=w332:string)  [unwired: 13 in]
      }
      frame "Macro: Sweeping" {
        # "Do not put any code in this frame.\n(It is a separator no-op. You can make a copy of this frame to create a new Macro frame)"
        n125 = call <vilib>:"Add State(s) to Queue__jki_lib_state_machine.vi"("State(s) in Front (\"\")"="Measure: Lockin\n//Measure: Temperature\nMeasure: Time\nMeasure: Delay Line\nUI: Update Graphs\nUI: Update Timer\nData: Reset >> False" ("State(s) in Front (\"\")"), "State(s) in (\"\")"=w338) -> ("States Out"=w337:string)  [unwired: 13 in]
      }
      frame "Macro: Stop Sweep" {
        # "Do not put any code in this frame.\n(It is a separator no-op. You can make a copy of this frame to create a new Macro frame)"
        n126 = call <vilib>:"Add State(s) to Queue__jki_lib_state_machine.vi"("State(s) in Front (\"\")"="//Sweep: Stop\nUI: Update Graphs Final\nFile: Save\n//Action: Lockin >> Stop" ("State(s) in Front (\"\")"), "State(s) in (\"\")"=w343) -> ("States Out"=w342:string)  [unwired: 13 in]
      }
      frame "Macro: Exit" {
        # "Exit Macro\n(This is called once, when the VI exits)"
        n127 = Unbundle By Name(w350) -> ("Core.Close Panel on Exit?"=w349:bool)
        n128 = Select(t="UI: Front Panel State >> Close", s=w349, f="") -> (s? t:f=w346:string)
        n129 = call <vilib>:"Add State(s) to Queue__jki_lib_state_machine.vi"("State(s) in (\"\")"=w346, "State(s) at Back (\"\")"="Data: Cleanup\nExit") -> ("States Out"=w344:string)  [unwired: 13 in]
        n130 = call <vilib>:"Add State(s) to Queue__jki_lib_state_machine.vi"("State(s) in Front (\"\")"=w344, "State(s) in (\"\")"=w353) -> ("States Out"=w352:string)  [unwired: 13 in]
      }
      frame "---------- Sweep ----------" {
        # "Do not put any code in this frame.\n(It is a separator no-op. You can make a copy of this frame to create a new Macro frame)"
        n131 = call <vilib>:"Add State(s) to Queue__jki_lib_state_machine.vi"("State(s) in (\"\")"=w357) -> ("States Out"=w356:string)  [unwired: 14 in]
      }
      frame "Sweep: Initialize" {
        # "Do not put any code in this frame.\n(It is a separator no-op. You can make a copy of this frame to create a new Macro frame)"
        n132 = Unbundle By Name(w369) -> ("Optical Delay Line"=w367)
        n133 = call-dynamic "Open.vi"("error in (no error)"=w366, "Instrument in"=w367) -> ("error out"=w362:errorcluster, "Instrument out"=w365:refnum<class "Instrument.DelayLine.lvclass">)  [unwired: 8 in]
        n134 = Subtract(x="Delay End (ps)", y="Delay Start (ps)") -> (x-y=w364:dbl)
        n135 = Absolute Value(x=w364) -> (abs(x)=w361:dbl)
        n136 = Divide(x=w361, y="Sweep Time (s)") -> (x/y=w363:dbl)
        n137 = property on="Horizontal Progress Bar" class="Slide (strict)"("Scale.Maximum"="Delay End (ps)", "Scale.Minimum"="Delay Start (ps)") -> ()  [unwired: 2 in, 2 out]
        n138 = Bundle By Name(cluster=w369, "Optical Delay Line"=w365, "Delay Range (ps)"=w361, "Delay Speed (ps/s)"=w363) -> (w368:T6)
        n139 = call <vilib>:"Add State(s) to Queue__jki_lib_state_machine.vi"("State(s) in (\"\")"=w371) -> ("States Out"=w370:string)  [unwired: 14 in]
      }
      frame "Sweep: Wait" {
        # "Do not put any code in this frame.\n(It is a separator no-op. You can make a copy of this frame to create a new Macro frame)"
        n140 = Multiply(x="Initial Wait (s)", y=u32 1000) -> (x*y=w373:u32)
        n141 = call <userlib>:"Wait (ms)__ogtk.vi"("error in (no error)"=w376, "milliseconds to wait"=w373) -> ("error out"=w375:errorcluster)  [unwired: 8 in, 1 out]
        n142 = call <vilib>:"Add State(s) to Queue__jki_lib_state_machine.vi"("State(s) in (\"\")"=w379) -> ("States Out"=w378:string)  [unwired: 14 in]
      }
      frame "Sweep: Stop" {
        # "#todo: is there a method to abort acquisition?"
        # "Do not put any code in this frame.\n(It is a separator no-op. You can make a copy of this frame to create a new Macro frame)"
        n143 = Unbundle By Name(w381) -> ()  [unwired: 1 out]
        n144 = call <vilib>:"Add State(s) to Queue__jki_lib_state_machine.vi"("State(s) in (\"\")"=w383) -> ("States Out"=w382:string)  [unwired: 14 in]
      }
      frame "Sweep: Check State" {
        # "Do not put any code in this frame.\n(It is a separator no-op. You can make a copy of this frame to create a new Macro frame)"
        n145 = Unbundle By Name(w389) -> ("delay line finish?"=w388:bool)
        n146 = Select(t="Macro: Sweeping\nMacro: Stop Sweep\nMacro: Exit" ("State(s) in Front (\"\")"), s=w388, f="") -> (s? t:f=w385:string)
        n147 = call <vilib>:"Add State(s) to Queue__jki_lib_state_machine.vi"("State(s) in Front (\"\")"=w385, "State(s) in (\"\")"=w391) -> ("States Out"=w390:string)  [unwired: 13 in]
      }
      frame "Sweep: Simulate" {
        # "Do not put any code in this frame.\n(It is a separator no-op. You can make a copy of this frame to create a new Macro frame)"
        n148 = Unbundle By Name(w393) -> ("Delay Speed (ps/s)"=w392:dbl)  [unwired: 1 out]
        n149 = while {
          tunnel: w392 -> [w406]
          i -> [w411]
          stop <- w409 stop-if-true
          n150 = Equal To 0?(x=w411) -> (x = 0?=w410:bool)
          n151 = local read "Delay Start (ps)"() -> (w408:dbl)
          n152 = call <userlib>:"MGI Milliseconds Since Last Reset.vi"("Reset (F)"=w410) -> ("ms"=w405:u32, "Error Out"=w399:errorcluster)  [unwired: 5 in]
          n153 = local read "Sweep Time (s)"() -> (w404:dbl)
          n154 = Divide(x=w405, y=1000.0) -> (x/y=w401:dbl)
          n155 = Multiply(x=w406, y=w401) -> (x*y=w402:dbl)
          n156 = call <userlib>:"MGI Milliseconds Since Last Call.vi"("Error In"=w399) -> ("ms"=w397:u32, "Error Out"=w398:errorcluster)  [unwired: 5 in]
          n157 = Add(x=w408, y=w402) -> (x+y=w407:dbl)
          n158 = local write "Elapsed Time (s)"(w401) -> ()
          n159 = Greater?(x=w401, y=w404) -> (0:w409:bool)
          n160 = local write "Refresh Time (ms)"(w397) -> ()
          n161 = call-poly <userlib>:"MGI Wait.vi"("ms"=u32 100, "Error In"=w398) -> ()  [unwired: 5 in, 1 out]
          n162 = local write "Horizontal Progress Bar"(w407) -> ()
          n163 = local write "Delay (ps)"(w407) -> ()
        }
        n164 = call <vilib>:"Add State(s) to Queue__jki_lib_state_machine.vi"("State(s) in (\"\")"=w396) -> ("States Out"=w395:string)  [unwired: 14 in]
      }
      frame "---------- Action ----------" {
        # "Do not put any code in this frame.\n(It is a separator no-op. You can make a copy of this frame to create a new Macro frame)"
        n165 = call <vilib>:"Add State(s) to Queue__jki_lib_state_machine.vi"("State(s) in (\"\")"=w415) -> ("States Out"=w414:string)  [unwired: 14 in]
      }
      frame "Action: Lockin" {
        # "Do not put any code in this frame.\n(It is a separator no-op. You can make a copy of this frame to create a new Macro frame)"
        n166 = Unbundle By Name(w416) -> ("Instruments.Lockin"=w419:refnum<class "Instrument.Lockin.lvclass">)
        n167 = case shown="\"Start\", Default" w420 {
          tunnel: w419 -> [w423 w438]
          tunnel: w418 -> [w424 w440]
          tunnel: [w425 w439] -> w417
          frame "Stop" {
            n168 = call <userlib>:"setIVmodeConfig.vi"("error in (no error)"=w424, "IV mode"=TRUE, "Instrument.Lockin in"=w423) -> ("error out"=w426:errorcluster, "Instrument.Lockin out"=w427:refnum<class "Instrument.Lockin.lvclass">)  [unwired: 7 in]
            n169 = while {
              shift-right: [w436] -> w425
              shift-left: w426 -> [w437]
              tunnel: w427 -> [w433]
              tunnel: [w432] -> _
              stop <- w434 stop-if-true
              n170 = call <userlib>:"Wait (ms)__ogtk.vi"("error in (no error)"=w437, "milliseconds to wait"=u32 100) -> ("error out"=w431:errorcluster)  [unwired: 8 in, 1 out]
              n171 = call <userlib>:"getStatus.vi"("error in (no error)"=w431, "Instrument.Lockin"=w433) -> ("error out"=w436:errorcluster, "Status"=w435:T9, "Instrument.Lockin"=w432:refnum<class "Instrument.Lockin.lvclass">)  [unwired: 7 in]
              n172 = Equal?(x=State-enum."idle" ("Status"), y=w435) -> (x = y?=w434:bool)
            }
          }
          frame "Start", Default {
            n173 = call <userlib>:"setIVmodeConfig.vi"("error in (no error)"=w440, "IV mode"=FALSE, "Instrument.Lockin in"=w438) -> ("error out"=w441:errorcluster, "Instrument.Lockin out"=w442:refnum<class "Instrument.Lockin.lvclass">)  [unwired: 7 in]
            n174 = while {
              shift-right: [w451] -> w439
              shift-left: w441 -> [w452]
              tunnel: w442 -> [w448]
              tunnel: [w447] -> _
              stop <- w449 stop-if-true
              n175 = call <userlib>:"Wait (ms)__ogtk.vi"("error in (no error)"=w452, "milliseconds to wait"=u32 100) -> ("error out"=w446:errorcluster)  [unwired: 8 in, 1 out]
              n176 = call <userlib>:"getStatus.vi"("error in (no error)"=w446, "Instrument.Lockin"=w448) -> ("error out"=w451:errorcluster, "Status"=w450:T9, "Instrument.Lockin"=w447:refnum<class "Instrument.Lockin.lvclass">)  [unwired: 7 in]
              n177 = Equal?(x=State-enum."started" ("Status"), y=w450) -> (x = y?=w449:bool)
            }
          }
        }
        n178 = call <vilib>:"Add State(s) to Queue__jki_lib_state_machine.vi"("State(s) in (\"\")"=w422) -> ("States Out"=w421:string)  [unwired: 14 in]
      }
      frame "Action: Lockin Sampling" {
        # "#todo: make sure Fs and N are in appropriate range"
        # "Do not put any code in this frame.\n(It is a separator no-op. You can make a copy of this frame to create a new Macro frame)"
        n179 = Unbundle By Name(w464) -> ("Instruments.Lockin"=w459:refnum<class "Instrument.Lockin.lvclass">)
        n180 = Multiply(x="Fs (S/s)", y="Lockin Refresh (s)") -> (x*y=w462:dbl)
        n181 = To Long Integer(number=w462) -> (32bit integer=w460:i32)
        n182 = call <userlib>:"getSampling.vi"("error in (no error)"=w456, "Instrument.Lockin in"=w459) -> ("error out"=w455:errorcluster, "sampling"=w453:T10, "Instrument.Lockin out"=w458:refnum<class "Instrument.Lockin.lvclass">)  [unwired: 7 in]
        n183 = Bundle By Name(cluster=w453, "Fs"="Fs (S/s)", "#s"=w460) -> (w454:T10)
        n184 = Not Equal?(x=w453, y=w454) -> (x != y?=w457:bool)
        n185 = case shown="True" w457 {
          tunnel: w455 -> [w468 w472]
          tunnel: [w468 w471] -> w465
          tunnel: w458 -> [_ w470]
          tunnel: w454 -> [_ w469]
          frame False {
          }
          frame True {
            n186 = call <userlib>:"setSampling.vi"("error in (no error)"=w472, "Sampling"=w469, "Instrument.Lockin in"=w470) -> ("error out"=w471:errorcluster)  [unwired: 7 in, 1 out]
          }
        }
        n187 = call <vilib>:"Add State(s) to Queue__jki_lib_state_machine.vi"("State(s) in (\"\")"=w467) -> ("States Out"=w466:string)  [unwired: 14 in]
      }
      frame "Action: Move Delay Line" {
        # "Do not put any code in this frame.\n(It is a separator no-op. You can make a copy of this frame to create a new Macro frame)"
        n188 = Unbundle By Name(w479) -> ("Optical Delay Line"=w480, "Delay Speed (ps/s)"=w477:dbl)
        n189 = case shown="\"End\"" w478 {
          tunnel: [w483 w486] -> w475
          tunnel: [1.0 ("Rate (ps/s)") w485] -> w476
          tunnel: w477 -> [_ w485]
          frame "Start", Default {
            n190 = local read "Delay Start (ps)"() -> (w483:dbl)
          }
          frame "End" {
            n191 = local read "Delay End (ps)"() -> (w486:dbl)
          }
        }
        n192 = call-dynamic "Set Delay.vi"("error in (no error)"=w474, "Rate (ps/s)"=w476, "Delay (ps)"=w475, "Instrument.Delay in"=w480) -> ("error out"=w473:errorcluster)  [unwired: 6 in, 1 out]
        n193 = call <vilib>:"Add State(s) to Queue__jki_lib_state_machine.vi"("State(s) in (\"\")"=w482) -> ("States Out"=w481:string)  [unwired: 14 in]
      }
      frame "Action: Close Delay Line" {
        # "Do not put any code in this frame.\n(It is a separator no-op. You can make a copy of this frame to create a new Macro frame)"
        n194 = Unbundle By Name(w490) -> ("Optical Delay Line"=w489)
        n195 = call-dynamic "Close.vi"("error in (no error)"=w488, "Instrument in"=w489) -> ("error out"=w487:errorcluster)  [unwired: 8 in, 1 out]
        n196 = call <vilib>:"Add State(s) to Queue__jki_lib_state_machine.vi"("State(s) in (\"\")"=w492) -> ("States Out"=w491:string)  [unwired: 14 in]
      }
      frame "---------- Measure ----------" {
        # "Template Separator\n(You can make a copy of, or modify, this frame)"
        n197 = call <vilib>:"Add State(s) to Queue__jki_lib_state_machine.vi"("State(s) in (\"\")"=w496) -> ("States Out"=w495:string)  [unwired: 14 in]
      }
      frame "Measure: Lockin" {
        # "Template Separator\n(You can make a copy of, or modify, this frame)"
        n198 = Unbundle By Name(w506) -> ("t0"=w499:timestamp, "AI Waveform (s)"=w504:waveform(dbl)[], "Instruments.Lockin"=w500:refnum<class "Instrument.Lockin.lvclass">)
        n199 = case shown="\"Start\"" w497 {
          tunnel: w504 -> [w512 w531]
          tunnel: [w512 w530] -> w503
          tunnel: [w514 w529] -> w502
          tunnel: w498 -> [w515 w528]
          tunnel: [w510 w524] -> w501
          tunnel: w500 -> [w516 w523]
          tunnel: w499 -> [_ w521]
          frame "Start" {
            n200 = for {
              N: 3 -> [_]
              tunnel: w516 -> [w520]
              tunnel: [w517] -> w509
              shift-right: [w518] -> w514
              shift-left: w515 -> [w519]
              n201 = call <userlib>:"waitForNewWaveforms.vi"("error in (no error)"=w519, "Instrument.Lockin in"=w520) -> ("error out"=w518:errorcluster, "Newest AI Waveform"=w517:waveform(dbl)[])  [unwired: 7 in, 1 out]
            }
            n202 = Index Array(array=w509) -> (element=w513:waveform(dbl))  [unwired: 1 in]
            n203 = Unbundle By Name(w513) -> ("t0"=w510:timestamp)
          }
          frame Default {
            n204 = call <userlib>:"getAIwfm.vi"("error in (no error)"=w528, "Instrument.Lockin in"=w523) -> ("error out"=w527:errorcluster, "AI Waveform"=w522:waveform(dbl)[])  [unwired: 7 in, 1 out]
            n205 = Index Array(array=w522) -> (element=w526:waveform(dbl))  [unwired: 1 in]
            n206 = Unbundle By Name(w526) -> ("t0"=w524:timestamp)
            n207 = Equal?(x=w524, y=w521) -> (x = y?=w525:bool)
            n208 = case shown="False" w525 {
              tunnel: w531 -> [w533 w550]
              tunnel: [w536 w550] -> w530
              tunnel: [w535 w551] -> w529
              tunnel: w527 -> [w534 w551]
              tunnel: w522 -> [w537 _]
              frame False {
                n209 = Array Size(array=w533) -> (size(s)=w532:i32)
                n210 = case shown="Default" w532 {
                  tunnel: w537 -> [w539 w544]
                  tunnel: [w539 w543] -> w536
                  tunnel: [w538 w542] -> w535
                  tunnel: w534 -> [w538 w541]
                  tunnel: w533 -> [_ w540]
                  frame 0 {
                  }
                  frame Default {
                    n211 = for {
                      tunnel: w540 -> [w545] mode=indexing
                      tunnel: w544 -> [w549] mode=indexing
                      tunnel: [w548] -> w543 mode=indexing
                      tunnel: [w547] -> w542
                      tunnel: w541 -> [w546]
                      n212 = call-poly <vilib>:"Append Waveforms.vi"("error in (no error)"=w546, "waveform B"=w549, "waveform A"=w545) -> ("error out"=w547:errorcluster, "waveform out"=w548:waveform(dbl))  [unwired: 7 in]
                    }
                  }
                }
              }
              frame True {
              }
            }
          }
        }
        n213 = Bundle By Name(cluster=w506, "t0"=w501, "AI Waveform (s)"=w503) -> (w505:T6)
        n214 = call <vilib>:"Add State(s) to Queue__jki_lib_state_machine.vi"("State(s) in (\"\")"=w508) -> ("States Out"=w507:string)  [unwired: 14 in]
      }
      frame "Measure: Temperature" {
        # "Your code here.\n(You can make a copy of, or modify, this frame)"
        n215 = Unbundle By Name(w559) -> ("Control Experiment"=w554:refnum<class "SMO.Control Experiment.lvclass">, "Instruments.Temperature"=w561:refnum<class "Instrument.Cryostat.lvclass">)
        n216 = call-dynamic "Get Temperature.vi"("error in (no error)"=w560, "Instrument.Cryostat in"=w561) -> ("error out"=w556:errorcluster, "Temperature (K)"=w555:dbl)  [unwired: 5 in, 3 out]
        "T (mK)" <- w555
        n217 = call "Append Dictionary Element.vi"("error in (no error)"=w556, "value"=w555, "key"="Temperature", "Control Experiment in"=w554) -> ("error out"=w553:errorcluster, "Control Experiment out"=w552:refnum<class "Control Experiment.lvclass">)  [unwired: 6 in]
        n218 = Bundle By Name(cluster=w559, "Control Experiment"=w552) -> (w558:T6)
        n219 = call <vilib>:"Add State(s) to Queue__jki_lib_state_machine.vi"("State(s) in (\"\")"=w563) -> ("States Out"=w562:string)  [unwired: 14 in]
      }
      frame "Measure: Time" {
        # "Your code here.\n(You can make a copy of, or modify, this frame)"
        n220 = Unbundle By Name(w582) -> ("reset"=w566:bool, "Elapsed Time"=w576:dbl[], "Absolute Time"=w570:dbl[], "Control Experiment"=w580:refnum<class "SMO.Control Experiment.lvclass">)
        n221 = Get Date/Time In Seconds() -> (seconds since 1Jan1904=w572:timestamp)
        n222 = Select(t=2, s=w566, f=1) -> (s? t:f=w567:i32)
        n223 = for {
          N: w567 -> [_]
          tunnel: [w587] -> w574
          tunnel: w566 -> [w586]
          n224 = call <userlib>:"MGI Milliseconds Since Last Reset.vi"("Reset (F)"=w586) -> ("ms"=w587:u32)  [unwired: 5 in, 1 out]
        }
        n225 = To Double Precision Float(number=w572) -> (double precision float=w569:dbl)
        n226 = Divide(x=w574, y=u32 1000) -> (x/y=w573:dbl)
        n227 = call "Append Dictionary Element.vi"("error in (no error)"=w578, "value"=w569, "key"="Time", "Control Experiment in"=w580) -> ("error out"=w577:errorcluster, "Control Experiment out"=w581:refnum<class "Control Experiment.lvclass">)  [unwired: 6 in]
        n228 = Build Array (concatenate)(w570, w569) -> (w571:dbl[])
        n229 = Build Array (concatenate)(w576, w573) -> (w575:dbl[])
        n230 = Bundle By Name(cluster=w582, "Elapsed Time"=w575, "Absolute Time"=w571, "Control Experiment"=w581) -> (w583:T6)
        n231 = call <vilib>:"Add State(s) to Queue__jki_lib_state_machine.vi"("State(s) in (\"\")"=w585) -> ("States Out"=w584:string)  [unwired: 14 in]
      }
      frame "Measure: Delay Line" {
        # "Template Separator\n(You can make a copy of, or modify, this frame)"
        n232 = Unbundle By Name(w600) -> ("Delay"=w594:dbl[], "Control Experiment"=w595:refnum<class "SMO.Control Experiment.lvclass">, "Optical Delay Line"=w598)
        n233 = call-dynamic "Get Delay.vi"("error in (no error)"=w592, "Instrument.Delay in"=w598) -> ("error out"=w596:errorcluster, "Delay (ps)"=w588:dbl, "Finished?"=w589:bool)  [unwired: 6 in, 1 out]
        "Delay (ps)" <- w588
        "Horizontal Progress Bar" <- w588
        n234 = Build Array (concatenate)(w594, w588) -> (w593:dbl[])
        n235 = call "Append Dictionary Element.vi"("error in (no error)"=w596, "value"=w588, "key"="Delay", "Control Experiment in"=w595) -> ("error out"=w591:errorcluster, "Control Experiment out"=w597:refnum<class "Control Experiment.lvclass">)  [unwired: 6 in]
        n236 = Bundle By Name(cluster=w600, "Delay"=w593, "Control Experiment"=w597, "delay line finish?"=w589) -> (w599:T6)
        n237 = call <vilib>:"Add State(s) to Queue__jki_lib_state_machine.vi"("State(s) in (\"\")"=w602) -> ("States Out"=w601:string)  [unwired: 14 in]
      }
      frame "---------- File ----------" {
        # "Template Separator\n(You can make a copy of, or modify, this frame)"
        n238 = call <vilib>:"Add State(s) to Queue__jki_lib_state_machine.vi"("State(s) in (\"\")"=w606) -> ("States Out"=w605:string)  [unwired: 14 in]
      }
      frame "File: Configure" {
        # "Template Separator\n(You can make a copy of, or modify, this frame)"
        n239 = call <vilib>:"Add State(s) to Queue__jki_lib_state_machine.vi"("State(s) in (\"\")"=w610) -> ("States Out"=w609:string)  [unwired: 14 in]
      }
      frame "File: Save" {
        # "Template Separator\n(You can make a copy of, or modify, this frame)"
        n240 = Unbundle By Name(w614) -> ("Execution:State"=w615:T7, "Control Experiment"=w616:refnum<class "SMO.Control Experiment.lvclass">, "AI Waveform (ps)"=w617:waveform(dbl)[])
        n241 = for {
          tunnel: w616 -> [w660]
          tunnel: [w659] -> w622
          tunnel: [w658] -> w621
          tunnel: w619 -> [w643]
          tunnel: w617 -> [w638] mode=indexing
          tunnel: w619 -> [w632]
          tunnel: [w625] -> w618 mode=indexing
          i -> [w665]
          n242 = call-poly <userlib>:"Waveform to XY.vi"("error in (no error)"=w632, "Waveform in"=w638) -> ("error out"=w633:errorcluster, "XY-data out"=w636:cluster{"X-array":dbl[], "Y-array":dbl[]})  [unwired: 8 in]
          n243 = call-poly <vilib>:"FFT Power Spectrum and PSD.vi"("error in (no error)"=w632, "time signal"=w638) -> ("error out"=w627:errorcluster, "Power Spectrum / PSD"=w625:cluster{"f0":dbl, "df":dbl, "magnitude":dbl[]})  [unwired: 6 in, 2 out]
          n244 = Increment(x=w665) -> (x+1=w663:i32)
          n245 = call-poly <userlib>:"Get X and Y.vi"("error in (no error)"=w633, "XY-data"=w636) -> ("Y-array"=w634:dbl[], "X-array"=w635:dbl[])  [unwired: 6 in, 2 out]
          n246 = Format Into String(format string="Ch%d" ("wavenames"), w663) -> (resulting string=w644:string)  [unwired: 2 in, 1 out]
          n247 = Unbundle By Name(w625) -> ("f0"=w642:dbl, "df"=w641:dbl, "magnitude"=w640:dbl[])
          n248 = Concatenate Strings(w644, "_x" ("string")) -> (w652:string)
          n249 = call "Write Dictionary Element.vi"("error in (no error)"=w643, "value"=w635, "key"=w652, "Control Experiment in"=w660) -> ("error out"=w656:errorcluster, "Control Experiment out"=w657:refnum<class "Control Experiment.lvclass">)  [unwired: 6 in]
          n250 = To Time Stamp(1:w642) -> (0:w639:timestamp)
          n251 = Concatenate Strings(w644, "_y" ("string")) -> (w650:string)
          n252 = Bundle By Name("t0"=w639, "dt"=w641, "Y"=w640) -> (w626:waveform(dbl))  [unwired: 1 in]
          n253 = call "Write Dictionary Element.vi"("error in (no error)"=w656, "value"=w634, "key"=w650, "Control Experiment in"=w657) -> ("error out"=w637:errorcluster, "Control Experiment out"=w662:refnum<class "Control Experiment.lvclass">)  [unwired: 6 in]
          n254 = Concatenate Strings(w644, "_PS" ("string")) -> (w647:string)
          n255 = call-poly <userlib>:"Waveform to XY.vi"("error in (no error)"=w627, "Waveform in"=w626) -> ("error out"=w631:errorcluster, "XY-data out"=w630:cluster{"X-array":dbl[], "Y-array":dbl[]})  [unwired: 8 in]
          n256 = call-poly <userlib>:"Get X and Y.vi"("error in (no error)"=w631, "XY-data"=w630) -> ("Y-array"=w628:dbl[], "X-array"=w629:dbl[])  [unwired: 6 in, 2 out]
          n257 = Concatenate Strings(w647, "_x" ("string")) -> (w646:string)
          n258 = call "Write Dictionary Element.vi"("error in (no error)"=w637, "value"=w629, "key"=w646, "Control Experiment in"=w662) -> ("error out"=w654:errorcluster, "Control Experiment out"=w655:refnum<class "Control Experiment.lvclass">)  [unwired: 6 in]
          n259 = Concatenate Strings(w647, "_y" ("string")) -> (w645:string)
          n260 = call "Write Dictionary Element.vi"("error in (no error)"=w654, "value"=w628, "key"=w645, "Control Experiment in"=w655) -> ("error out"=w658:errorcluster, "Control Experiment out"=w659:refnum<class "Control Experiment.lvclass">)  [unwired: 6 in]
        }
        "Power Spectrum" <- w618
        n261 = call "Exec State to Append.vi"("Execution:State"=w615) -> ("append?"=w611:bool)  [unwired: 2 in]
        n262 = call "Save Transport TDMS File.vi"("error in (no error)"=w621, 10:w611, "Control Experiment in"=w622) -> ("error out"=w620:errorcluster, "Control Experiment out"=w612:refnum<class "Control Experiment.lvclass">)  [unwired: 7 in]
        n263 = Bundle By Name(cluster=w614, "Control Experiment"=w612) -> (w613:T6)
        n264 = call <vilib>:"Add State(s) to Queue__jki_lib_state_machine.vi"("State(s) in (\"\")"=w624) -> ("States Out"=w623:string)  [unwired: 14 in]
      }
      frame "File: JSON" {
        # "#todo: add save JSON stuff"
        # "Template Separator\n(You can make a copy of, or modify, this frame)"
        n265 = Unbundle By Name(w667) -> ()  [unwired: 1 out]
        n266 = call <vilib>:"Add State(s) to Queue__jki_lib_state_machine.vi"("State(s) in (\"\")"=w669) -> ("States Out"=w668:string)  [unwired: 14 in]
      }
    }
  }
  "error out" <- w3
  n267 = Unbundle By Name(w4) -> ("Transport"=→"Transport out":refnum<class "SMO.Transport.lvclass">)
